vi "ENVIA VALORES-CLIENTE.vi"() -> ()   [LabVIEW 2019]
panel:
  out "Pfundo[kPa]":dbl
  in  "ValoresEnviados":cluster{"Pfundo[kPa]":dbl}
  out "size(s)":i32
  in  "stop":bool
  in  "VALORES VAZIOS":string[](array[string])
  out "RAN":dbl
  in  "FRA":string
  in  "FLO":dbl
  in  "NUM":i32
  in  "BOTAO":bool
  in  "NOMES":string[](array[string])
  out "Controles":cluster{refnum<vi>[]}
  out "VALORES":string[](array[string])
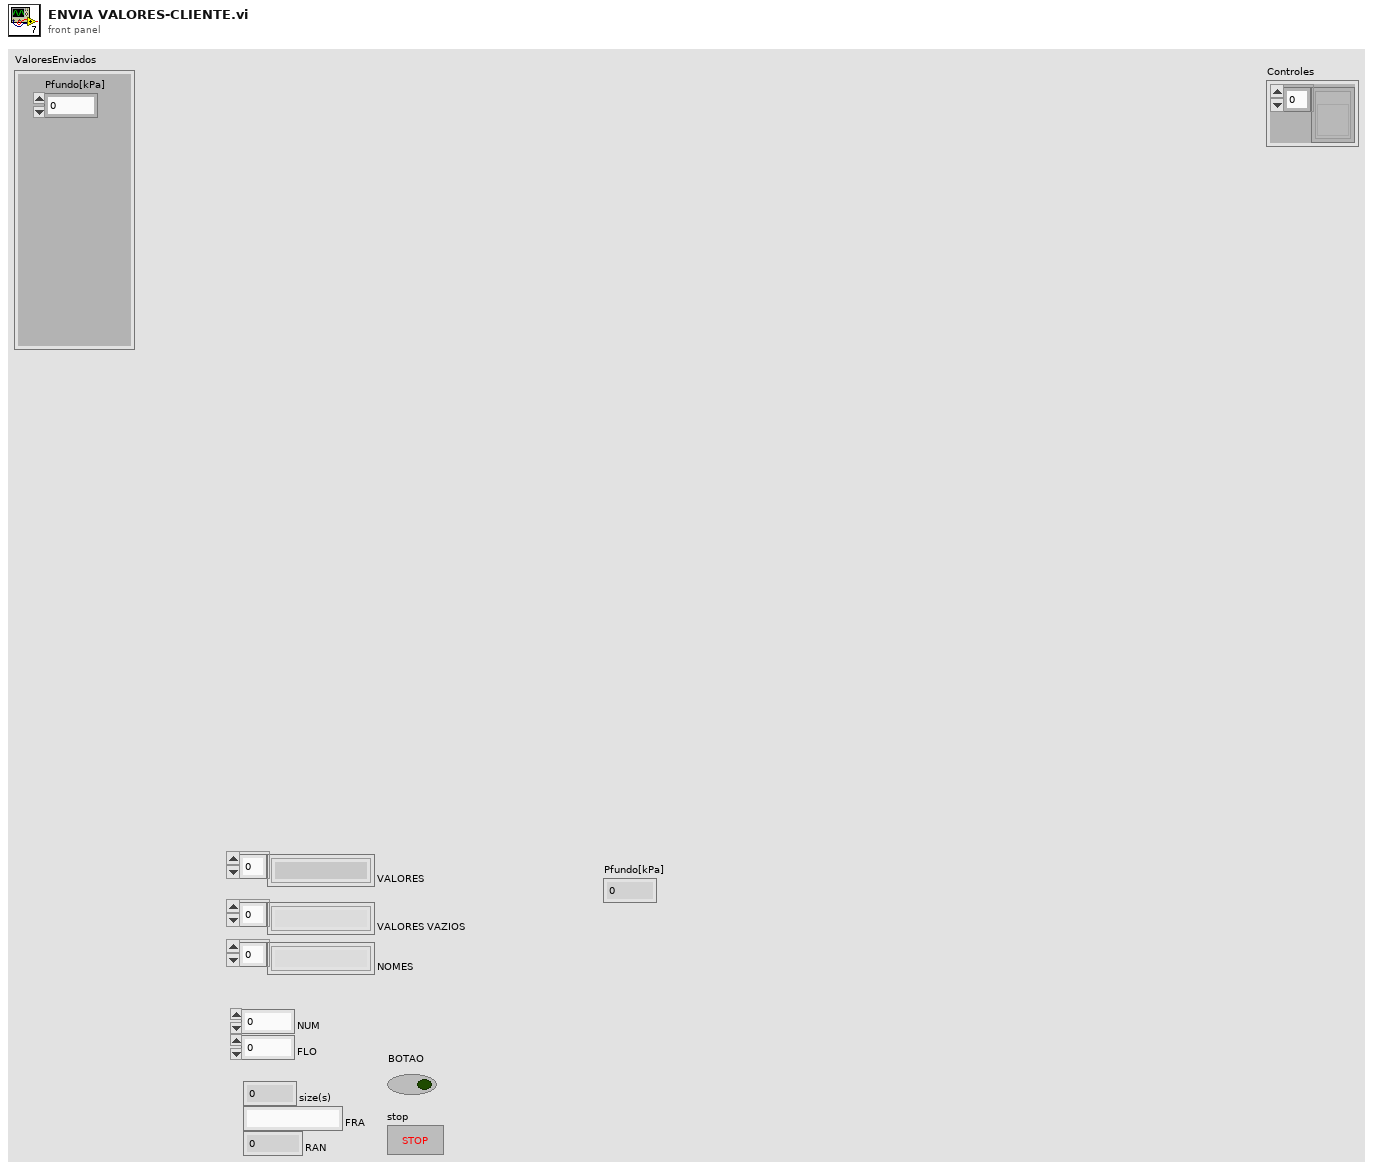
[diagram p1: front panel]
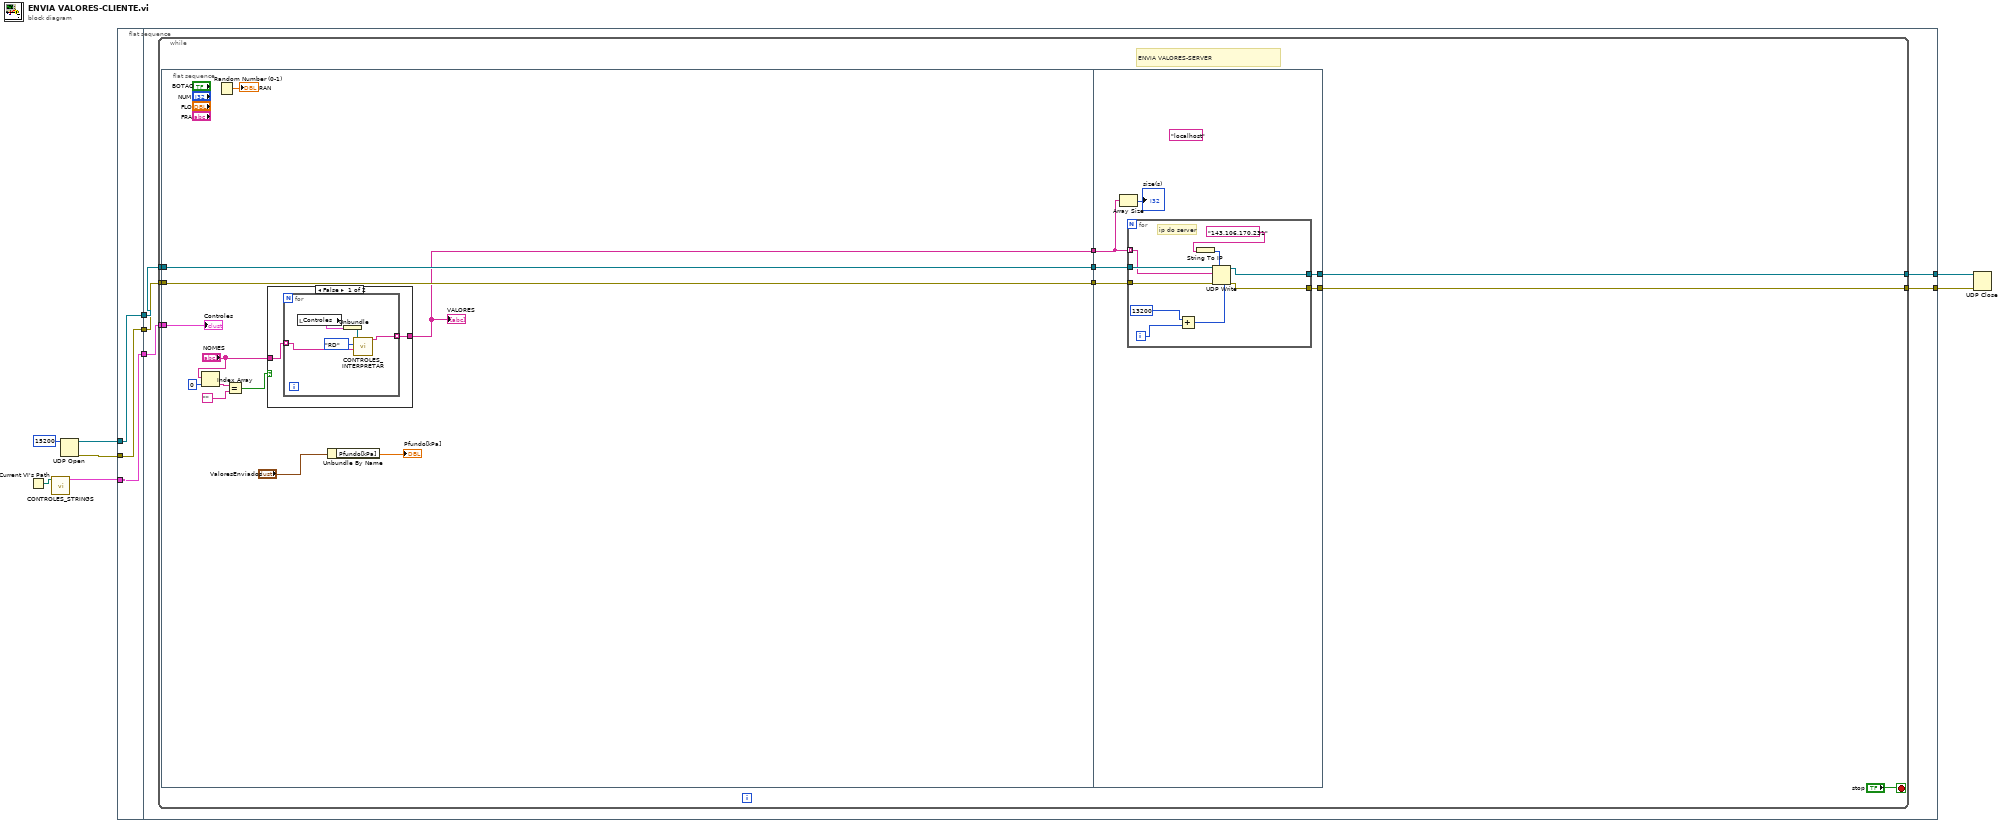
[diagram p0: block diagram]
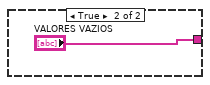
[diagram p2: hidden frame]
diagram:
  n1 = Current VI's Path() -> (path=w7:path)
  n2 = call "CONTROLES_STRINGS.vi"("vi path"=w7) -> ("output cluster"=w6:cluster{refnum<vi>[]})  [unwired: 9 in, 1 out]
  n3 = UDP Open(11:u16 15200 ("port")) -> (port=w9:refnum<k16>, 0:w8:errorcluster)  [unwired: 4 in, 1 out]
  n4 = flat-sequence {
    tunnel: w6 -> [w11]
    tunnel: w8 -> [w12]
    tunnel: w9 -> [w13]
    tunnel: [w13] -> w5
    tunnel: [w12] -> w4
    tunnel: [w11] -> w3
    tunnel: w5 -> [w15]
    tunnel: w4 -> [w14]
    tunnel: w3 -> [w18]
    tunnel: [w17] -> w2
    tunnel: [w16] -> w1
    frame #0 {
    }
    frame #1 {
      n5 = while {
        tunnel: w18 -> [w27]
        tunnel: [w25] -> w17
        tunnel: [w24] -> w16
        tunnel: w15 -> [w23]
        tunnel: w14 -> [w22]
        stop <- "stop" stop-if-true
        # "ENVIA VALORES-SERVER"
        n6 = flat-sequence {
          tunnel: [w39] -> w21
          tunnel: [w38] -> w20
          tunnel: [w37] -> w19
          tunnel: w23 -> [w39]
          tunnel: w22 -> [w38]
          tunnel: w27 -> [w35]
          tunnel: [w51] -> w25
          tunnel: [w50] -> w24
          tunnel: w21 -> [w53]
          tunnel: w20 -> [w52]
          tunnel: w19 -> [w49]
          frame #0 {
            n7 = Index Array(array="NOMES", index=0) -> (element=w32:string)
            n8 = Random Number (0-1)() -> (number: 0 to 1=→"RAN":dbl)
            n9 = Equal?(x=w32, y="") -> (x = y?=w30:bool)
            n10 = case shown="False" w30 {
              tunnel: [w41 "VALORES VAZIOS"] -> w37
              tunnel: "NOMES" -> [w40 _]
              frame False {
                n11 = for {
                  tunnel: w40 -> [w44] mode=indexing
                  tunnel: [w42] -> w41 mode=indexing
                  n12 = local read "Controles"() -> (w46:cluster{refnum<vi>[]})
                  n13 = Unbundle(w46) -> (w45:refnum<vi>[])
                  n14 = call "CONTROLES_INTERPRETAR.vi"("name"=w44, "RD/WR"=enum16{"WR", "RD"}."RD", "Controls[]"=w45) -> ("Data"=w42:string)  [unwired: 6 in, 2 out]
                }
              }
              frame True {
              }
            }
            "VALORES" <- w37
            n15 = Unbundle By Name("ValoresEnviados") -> ("Pfundo[kPa]"=→"Pfundo[kPa]":dbl)
            "Controles" <- w35
          }
          frame #1 {
            (unwired) "localhost" ("name")
            n16 = Array Size(array=w49) -> (size(s)=→"size(s)":i32)
            n17 = for {
              tunnel: w53 -> [w63]
              tunnel: w52 -> [w62]
              tunnel: w49 -> [w57] mode=indexing
              tunnel: [w56] -> w51
              tunnel: [w55] -> w50
              i -> [w60]
              # "ip do server"
              n18 = Add(x=u16 13200 ("port or service name"), y=w60) -> (x+y=w58:i32)
              n19 = String To IP(1:"143.106.170.231" ("name")) -> (0:w61:u32)
              n20 = UDP Write(address=w61, port or service name=w58, connection ID=w63, data in=w57, 8:w62) -> (error out=w55:errorcluster, 3:w56:refnum<k16>)  [unwired: 1 in]
            }
          }
        }
      }
    }
  }
  n21 = UDP Close(connection ID=w2, 8:w1) -> ()  [unwired: 2 out]
